vi "Get_Cluster_Argument.vi"(1 "source":refnum<vi>, 2 "Prefix":string, 3 "Argument List In":string[](array[string])) -> (0 "Argument List Out":string[](array[string]))   [LabVIEW 2011]
doc: "This VI parses an argument to find it's text value. For example, given an argument in the form of Arg(\"some text\"), it would return \"some text\", without quotation marks."
panel:
  out "concatenated string":string
  out "error out":errorcluster
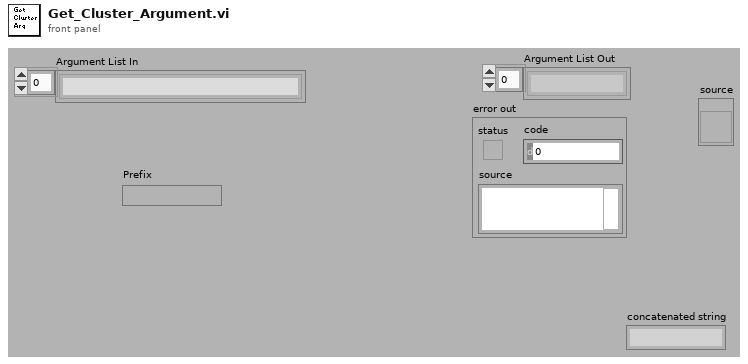
[diagram p1: front panel]
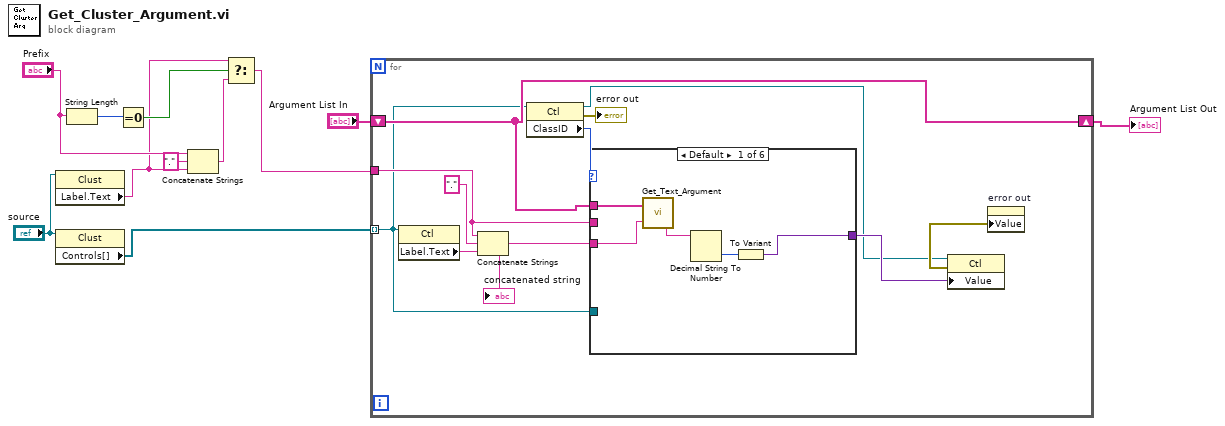
[diagram p0: block diagram]
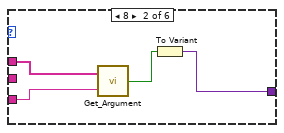
[diagram p2: hidden frame]
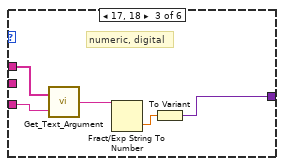
[diagram p3: hidden frame]
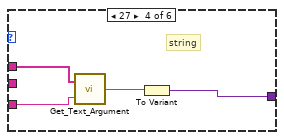
[diagram p4: hidden frame]
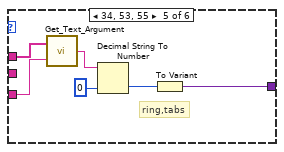
[diagram p5: hidden frame]
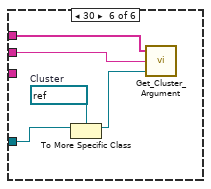
[diagram p6: hidden frame]
diagram:
  n1 = property class="Clust"(reference="source") -> ("Label.Text"=w2:string)  [unwired: 1 in, 2 out]
  n2 = property class="Clust"(reference="source") -> ("Controls[]"=w9:refnum<vi>[])  [unwired: 1 in, 2 out]
  n3 = String Length(string="Prefix") -> (length=w7:i32)
  n4 = Equal To 0?(x=w7) -> (x = 0?=w6:bool)
  n5 = Concatenate Strings("Prefix", "." ("string"), w2) -> (w3:string)
  n6 = Select(t=w2, s=w6, f=w3) -> (s? t:f=w1:string)
  n7 = for {
    tunnel: w9 -> [w12] mode=indexing
    shift-right: [w15] -> w10
    shift-left: "Argument List In" -> [w15]
    tunnel: w1 -> [w13]
    n8 = property class="Ctl"(reference=w12) -> ("Label.Text"=w20:string)  [unwired: 1 in, 2 out]
    n9 = Concatenate Strings(w13, "." ("string"), w20) -> (w14:string)
    "concatenated string" <- w14
    n10 = property class="Ctl"(reference=w12) -> (reference out=w16:refnum<vi>, error out=→"error out":errorcluster, "ClassID"=w22:u32)  [unwired: 1 in]
    n11 = case shown="Default" w22 {
      tunnel: [w26 w31 w35 w40 w44 _] -> w17
      tunnel: w15 -> [w25 w29 w33 w38 w42 w50]
      tunnel: w14 -> [w24 w30 w34 w37 w43 _]
      tunnel: w13 -> [_ _ _ _ _ w51]
      tunnel: w12 -> [_ _ _ _ _ w49]
      frame Default {
        n12 = call "Get_Text_Argument.vi"("Argument"=w24, "Argument List"=w25) -> ("Text"=w23:string)
        n13 = Decimal String To Number(string=w23) -> (number=w27:i32)  [unwired: 2 in, 1 out]
        n14 = To Variant(anything=w27) -> (Variant=w26:variant)
      }
      frame 8 {
        n15 = call "Get_Argument.vi"("Argument"=w30, "Argument List"=w29) -> ("Enabled"=w28:bool)
        n16 = To Variant(anything=w28) -> (Variant=w31:variant)
      }
      frame 17, 18 {
        # "numeric, digital"
        n17 = call "Get_Text_Argument.vi"("Argument"=w34, "Argument List"=w33) -> ("Text"=w32:string)
        n18 = Fract/Exp String To Number(string=w32) -> (number=w36:dbl)  [unwired: 3 in, 1 out]
        n19 = To Variant(anything=w36) -> (Variant=w35:variant)
      }
      frame 27 {
        # "string"
        n20 = call "Get_Text_Argument.vi"("Argument"=w37, "Argument List"=w38) -> ("Text"=w39:string)
        n21 = To Variant(anything=w39) -> (Variant=w40:variant)
      }
      frame 34, 53, 55 {
        # "ring,tabs"
        n22 = call "Get_Text_Argument.vi"("Argument"=w43, "Argument List"=w42) -> ("Text"=w41:string)
        n23 = Decimal String To Number(string=w41, default (0L)=u16 0 ("default (0 I32)")) -> (number=w46:u16)  [unwired: 1 in, 1 out]
        n24 = To Variant(anything=w46) -> (Variant=w44:variant)
      }
      frame 30 {
        w48 = refnum<vi> refnum  # Cluster
        n25 = To More Specific Class(target class=w48, reference=w49) -> (specific class reference=w47:refnum<vi>)  [unwired: 1 in, 1 out]
        n26 = call "Get_Cluster_Argument.vi"("source"=w47, "Prefix"=w51, "Argument List In"=w50) -> ()  [unwired: 1 out]
      }
    }
    n27 = property class="Ctl"(reference=w16, "Value"=w17) -> (error out=w18:errorcluster)  [unwired: 1 in, 1 out]
    n28 = property on="error out" class="Clust (strict)"("Value"=w18) -> ()  [unwired: 2 in, 2 out]
  }
  "Argument List Out" <- w10
